vi "Arm_GaGe4.vi"(0 "GaGe settings":cluster{"Mode":u16}={"Mode"=1} {"Mode" items=["Single", "Dual", "Quad", "Octal"]}, 1 "Handle Cluster":T1, 5 "Timing":T3 {"Pre-trigger length" format="%#_4p"; "Record length" format="%#_6p"; "Data rate" format="%#_6p"}, 7 "Input settings":T5(array[cluster]), 9 "Device":T2, 11 "error in (no error)":errorcluster, 12 "Trigger and sampling":T4={"Trig. edge"=enum."Falling", "Trig. type"=enum."Reference", "Trig. level"=2.0, "Average samples"=TRUE, "Oversample\nto match rates"=FALSE} {"Trig. level" format="%.2f"}) -> (2 "Triggered":bool, 3 "Armed":bool, 4 "GaGe settings out":cluster{"Mode":u16}={"Mode"=1} {"Mode" items=["Single", "Dual", "Quad", "Octal"]}, 6 "Timing":T3 {"Pre-trigger length" format="%#_4p"; "Record length" format="%#_6p"; "Data rate" format="%#_6p"}, 8 "Input settings out":T5(array[cluster]), 10 "Device out":T2, 13 "Parameters":string, 14 "Complete":bool, 15 "error out":errorcluster)   [LabVIEW 2015]
doc: "DESCRIPTION:\nThis VI retrieves the specified amount of data from one or more analog input channels each time a digital start trigger, digital stop trigger, or digital start and stop trigger, occur. It shows how to trigger an acquisition multiple times while avoiding the overhead of configuration and buffer allocation each time. This is a timed acquisition, meaning that a hardware clock is used to control the acquisition rate for fast and accurate timing. It is also a buffered acquisition, meaning that the data are stored in an intermediate memory buffer after they are acquired from the DAQ board. When the pretrigger scans is set to 0, you must set \"choose trigger type\" to START OR STOP TRIGGER (and use a start trigger). Your start trigger will then start your DAQ board and acquisition into a buffer to be read by LabVIEW. When the pretrigger scans is set to greater than 1, you can set \"choose trigger type\" to START OR STOP TRIGGER (and use a stop trigger) or START & STOP TRIGGER (and use both). If you use only the stop trigger, a software strobe starts your DAQ board and your stop trigger will determine when data are acquired into a buffer to be read by LabVIEW. If you use a start and stop trigger, your start trigger will start the DAQ board, but your stop trigger will determine when data are acquired into a buffer to be read by LabVIEW. In either case, your pretrigger scans will be the number of scans to acquire before the stop trigger occurs. The rest of the number of scans to acquire will be after the stop trigger. Data are retrieved from that buffer and displayed after the appropriate amount (before and after the stop trigger) have been acquired. The vertical cursor on the graph indicates where the trigger occurred. With each iteration of the while loop, the VI waits for the next trigger, then reads the same amount of data again from the same channels at the same rate.\n\nUse this VI to wait for multiple digital triggers, acquiring a relatively small amount of data for each trigger (it must fit in the memory available), where each point does not need to be viewed or processed while it is being acquired\n\nINSTRUCTIONS:\n1. Enter the device number, channels, number of scans to acquire, and scan rate.\n2. Enter the pretrigger scans, trigger edge, and time limit.\n3. Set choose trigger type to START OR STOP TRIGGER (to hardware start) if pretrigger scans = 0, If pretrigger scans > 0, set it to START OR STOP TRIGGER (to software start and hardware stop) or START & STOP TRIGGER (to hardware start and hardware stop).\n4. Make the appropriate I/O connections as explained below.\n5. Run the VI.\n\nKEY PARAMETERS:\nThis VI shows how to use the intermediate analog input DAQ VIs to trigger multiple acquisitions. \n\nAI Config.vi is only called on the first iteration of the while loop. This avoids the overhead of configuration and buffer allocation for each acquisition. However, you must stop and restart the VI if you wish to change input parameters.\n\nThe \"read/search mode\" for AI Read.vi is set to \"relative to trigger point\", since this is a hardware triggered acquisition. \n\nAI Control.vi (an advanced analog input VI) is called, in the event that AI Read.vi times out, to momentarily stop the analog input clock. This is needed so the input clock is not running when AI Start.vi (which restarts the clock) is called again.\n\nI/O CONNECTIONS:\nConnect to the input channels on the I/O connector for your board to match the channels you have chosen on the front panel of this VI. For example ACH0 for analog input.\n\nE series boards:\nConnect your start trigger to PFI0/TRIG1, your stop trigger to PFI1/TRIG2.\n\nLegacy MIO boards:\nConnect your start trigger to STARTRIG*, your stop trigger to STOPTRIG.\n\nLegacy MIO-16X, MIO-16F-5, and MIO-64F-5:\nThe start and stop trigger pin is EXTTRIG*.\n\nLab/1200 series boards:\nConnect your start or stop trigger to EXTTRIG. Hardware pretriggering (start & stop) is not supported.\n\nThe PC-LPM-16, DAQCard-500, and DAQCard-700 are not supported by this example.\n\nTo find the actual pin numbers, refer to your hardware user manual.\n\nDAQ VIs USED:\nAI Config.vi, AI Start.vi, AI Read.vi, AI Control.vi, AI Clear.vi."
uses:
  Utilities/Controls/Timing Element.ctl
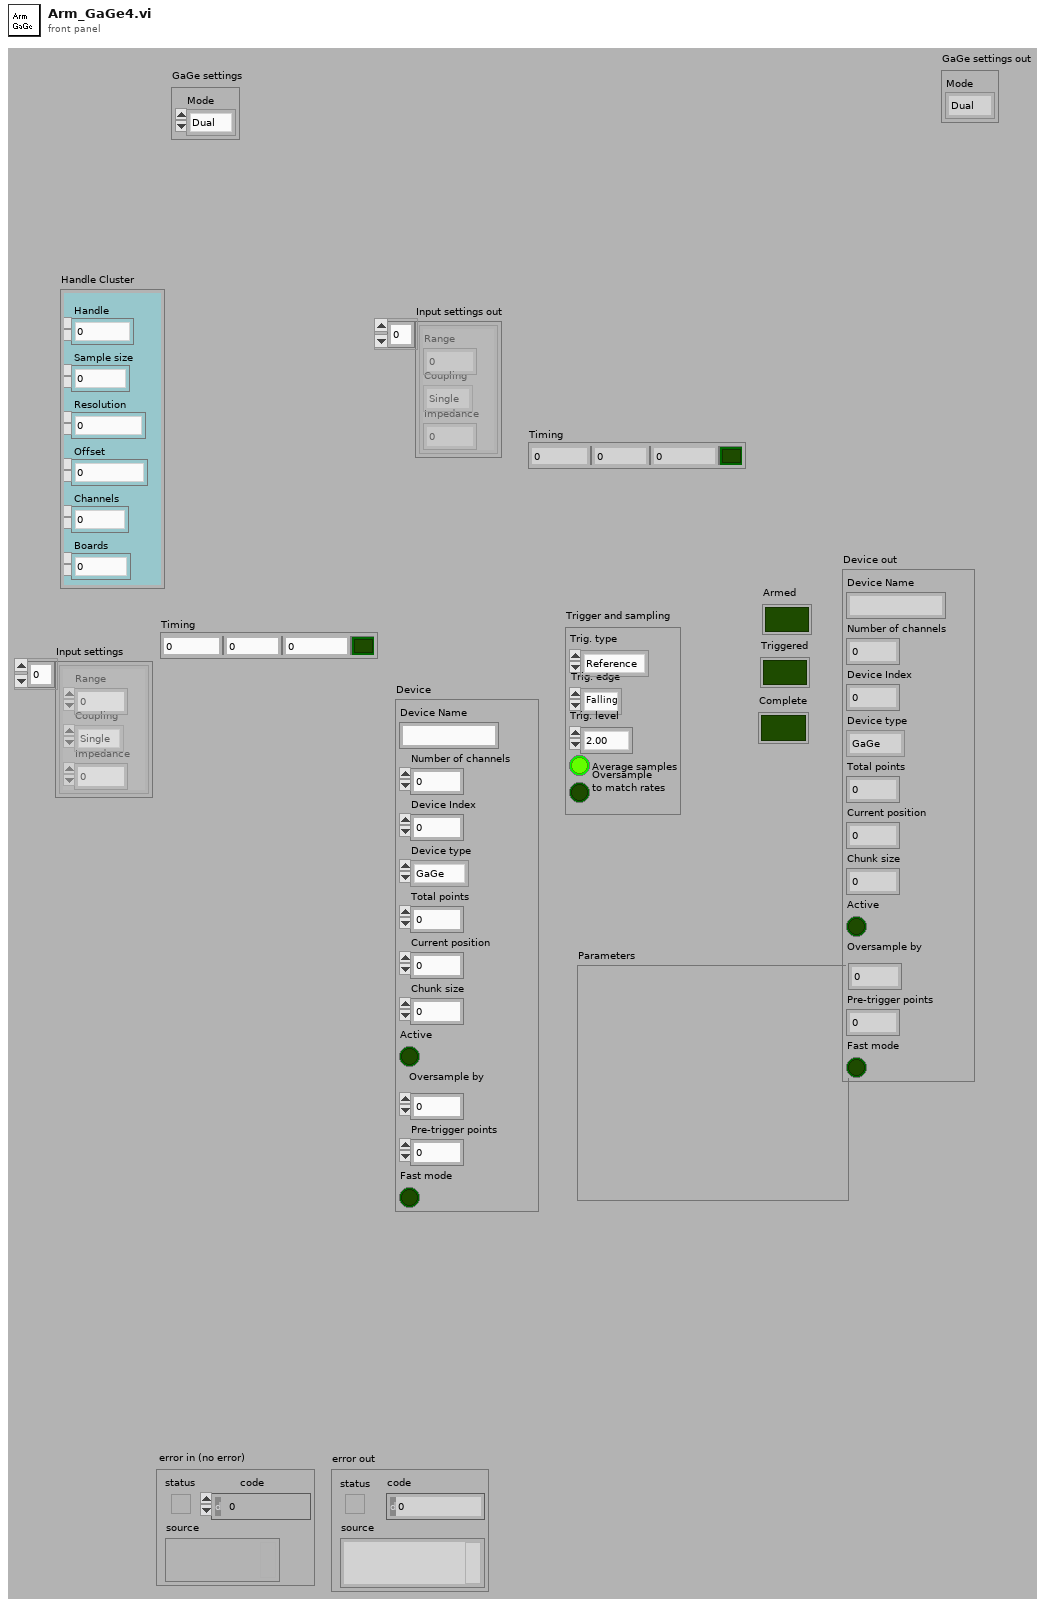
[diagram p1: front panel]
types:
  T1 = cluster{"Handle":u32, "Sample size":u32, "Resolution":i32, "Offset":i32, "Channels":u32, "Boards":u32}
  T2 = cluster{"Device Name":string, "Number of channels":i32, "Device Index":i32, "Device type":enum16{"GaGe", "NI-DAQ", "NI-Scope", "CAMAC", "VXI-1433", "VXI-1437"}, "Total points":i64, "Current position":i64, "Chunk size":i64, "Active":bool, "Oversample by":i32, "Pre-trigger points":i64, "Fast mode":bool}
  T3 = typedef "Timing Element.ctl" = cluster{"Data rate":dbl, "Record length":dbl, "Pre-trigger length":dbl, "Ext. clock":bool}
  T4 = cluster{"Trig. edge":enum16{"Rising", "Falling"}, "Trig. type":enum16{"Reference", "Immediate", "Start"}, "Trig. level":sgl, "Average samples":bool, "Oversample\nto match rates":bool}
  T5 = cluster{"Range":dbl, "Coupling":enum16{"Single", "Differen"}, "Impedance":dbl}[]
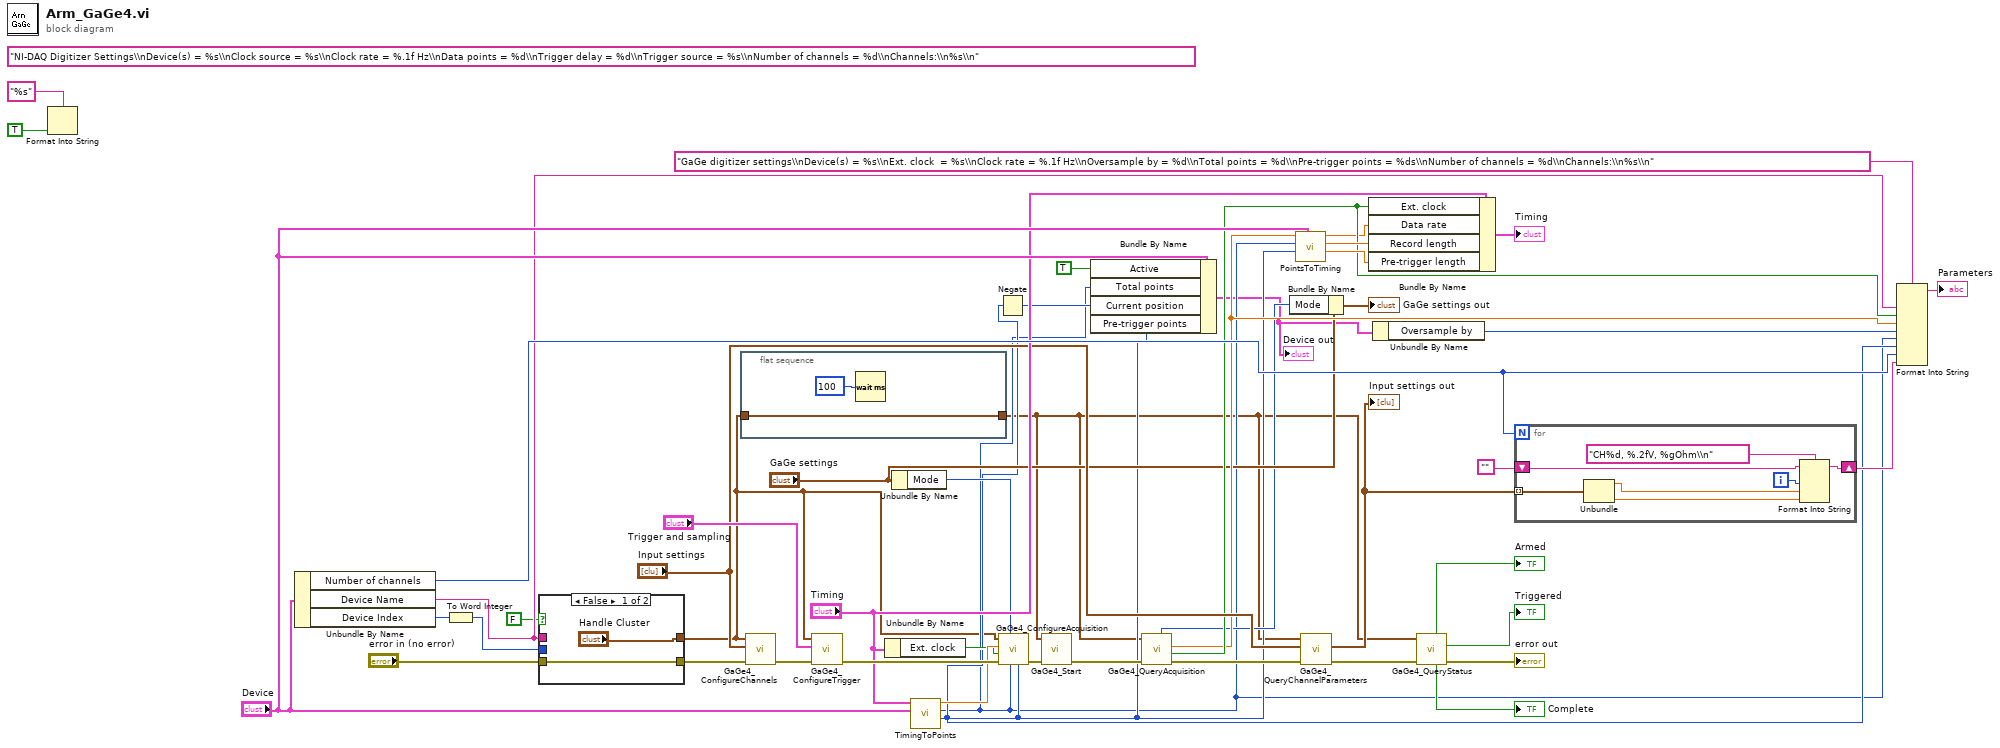
[diagram p0: block diagram]
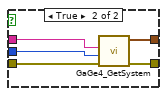
[diagram p2: hidden frame]
diagram:
  (unwired) "NI-DAQ Digitizer Settings\\nDevice(s) = %s\\nClock source = %s\\nClock rate = %.1f Hz\\nData points = %d\\nTrigger delay = %d\\nTrigger source = %s\\nNumber of channels = %d\\nChannels:\\n%s\\n" ("Format String")
  n1 = Format Into String(format string="%s", TRUE) -> ()  [unwired: 2 in, 2 out]
  n2 = Unbundle By Name("Device") -> ("Number of channels"=w40:i32, "Device Name"=w36:string, "Device Index"=w13:i32)
  n3 = To Word Integer(number=w13) -> (16bit integer=w12:i16)
  n4 = case shown="False" FALSE {
    tunnel: "error in (no error)" -> [w49 w55]
    tunnel: w36 -> [_ w54]
    tunnel: [w49 w53] -> w35
    tunnel: ["Handle Cluster" w52] -> w2
    tunnel: w12 -> [_ w51]
    frame False {
    }
    frame True {
      n5 = call "GaGe4_GetSystem.vi"("error in (no error)"=w55, "Board index"=w51, "Board Name (Any)"=w54) -> ("error out"=w53:errorcluster, "Handle Cluster out"=w52:T1)  [unwired: 7 out]
    }
  }
  n6 = flat-sequence {
    tunnel: w2 -> [w57]
    tunnel: [w57] -> w1
    frame #0 {
      n7 = Wait (ms)(milliseconds to wait=u32 100) -> ()  [unwired: 1 out]
    }
  }
  n8 = call "GaGe4_ConfigureChannels.vi"("error in (no error)"=w35, "Input settings"="Input settings", "Handle Cluster in"=w2) -> ("error out"=w34:errorcluster)  [unwired: 8 out]
  n9 = call "GaGe4_ConfigureTrigger.vi"("error in (no error)"=w34, "Trigger and sampling"="Trigger and sampling", "Handle Cluster in"=w2) -> ("error out"=w32:errorcluster)  [unwired: 8 out]
  n10 = Unbundle By Name("Timing") -> ("Ext. clock"=w29:bool)
  n11 = Unbundle By Name("GaGe settings") -> ("Mode"=w28:u16)
  n12 = call "TimingToPoints.vi"("Device"="Device", "Timing"="Timing") -> ("Pre-trigger points"=w10:i64, "Total points"=w9:i64, "Actual Rate, Hz"=w31:dbl)  [unwired: 7 out]
  n13 = Negate(x=w10) -> (-x=w11:i64)
  n14 = call "GaGe4_ConfigureAcquisition .vi"("Pre-trigger points"=w10, "Total points"=w9, "Mode"=w28, "error in (no error)"=w32, "Ext. clock"=w29, "Sample Rate"=w31, "Handle Cluster in"=w2) -> ("error out"=w27:errorcluster)  [unwired: 4 out]
  n15 = call "GaGe4_Start.vi"("error in (no error)"=w27, "Handle Cluster"=w1) -> ("error out"=w14:errorcluster)  [unwired: 9 out]
  n16 = Bundle By Name(cluster="Device", "Active"=TRUE, "Total points"=w9, "Current position"=w11, "Pre-trigger points"=w10) -> (w5:T2)
  "Device out" <- w5
  n17 = call "GaGe4_QueryAcquisition .vi"("error in (no error)"=w14, "Handle Cluster in"=w1) -> ("error out"=w26:errorcluster, "Ext. clock"=w21:bool, "Sample Rate"=w19:dbl, "Mode"=w17:u16)  [unwired: 6 out]
  n18 = Bundle By Name(cluster="GaGe settings", "Mode"=w17) -> (→"GaGe settings out":cluster{"Mode":u16})
  n19 = call "PointsToTiming.vi"("Device"="Device", "Pre-trigger points"=w10, "Total points"=w9, "Actual Rate, Hz"=w19) -> ("Pre-trigger length, s"=w42:dbl, "Record length, s"=w43:dbl, "Data rate, Hz"=w20:dbl)  [unwired: 2 in, 3 out]
  n20 = call "GaGe4_QueryChannelParameters .vi"("error in (no error)"=w26, "Input settings"="Input settings", "Handle Cluster in"=w1) -> ("error out"=w15:errorcluster, "Input settings out"=w24:T5)  [unwired: 7 out]
  "Input settings out" <- w24
  n21 = Bundle By Name(cluster="Timing", "Ext. clock"=w21, "Data rate"=w20, "Record length"=w43, "Pre-trigger length"=w42) -> (→"Timing":T3)
  n22 = Unbundle By Name(w5) -> ("Oversample by"=w4:i32)
  n23 = call "GaGe4_QueryStatus.vi"("error in (no error)"=w15, "Handle Cluster"=w1) -> ("error out"=→"error out":errorcluster, "Triggered"=→"Triggered":bool, "Complete"=→"Complete":bool, "Armed"=→"Armed":bool)  [unwired: 1 in, 5 out]
  n24 = for {
    N: w40 -> [_]
    tunnel: w24 -> [w64] mode=indexing
    shift-right: [w61] -> w44
    shift-left: "" -> [w62]
    i -> [w58]
    n25 = Unbundle(w64) -> ("Range"=w60:dbl, "Impedance"=w59:dbl)  [unwired: 1 out]
    n26 = Format Into String(format string="CH%d, %.2fV, %gOhm\\n", initial string=w62, w58, w60, w59) -> (resulting string=w61:string)  [unwired: 1 in, 1 out]
  }
  n27 = Format Into String(format string="GaGe digitizer settings\\nDevice(s) = %s\\nExt. clock  = %s\\nClock rate = %.1f Hz\\nOversample by = %d\\nTotal points = %d\\nPre-trigger points = %ds\\nNumber of channels = %d\\nChannels:\\n%s\\n" ("Format String"), w36, w21, w19, w4, w9, w10, w40, w44) -> (resulting string=→"Parameters":string)  [unwired: 2 in, 1 out]
